vi "Create DatabaseTable.vi"() -> ()   [LabVIEW 2018]
doc: "This example allows you to perform several tasks on a database named LabVIEW.mdb located in the LabVIEW examples>>database directory.\n\nOperations include creating a table, creating a table and inserting data into named fields, creating a table and inserting data into generically named fields, or deleting a table."
uses:
  <vilib>/addons/database/Auxilliary.llb/DB Tools Column Info.ctl
  <vilib>/addons/database/Auxilliary.llb/DB Tools DataTypes.ctl
  <vilib>/addons/database/Connection.llb/DB Tools Open Connec (Path).vi
  <vilib>/addons/database/NI_Database_API.lvlib
panel:
  in  "sample data":T1={"String"="This is a test string", "Numeric"=101, "Numeric 2"=3.14}
  in  "column information":T2[](array[typedef])=[{"column name"="stringcol", "data type"=enum."String", "size"=50, "allow null?"=FALSE}, {"column name"="intcol", "data type"=enum."Long (I32)", "size"=0, "allow null?"=TRUE}, {"column name"="doublecol", "data type"=enum."Double (DBL)", "size"=0, "allow null?"=TRUE}]
  in  "Function":u16(ring) items=["Create Only", "Create and Insert (With Names)", "Create and Insert (Generic Names)", "Delete Table"]
  in  "Table":string="createtable"
  # "Overview: Demonstrates how to perform several tasks on a database.\nRequirements: Database Connectivity Toolkit\nInstructions:\n1. Select one of the 'Create' operations in the Function ring.\n2. Run the VI. The database table will be updated.\n3. Select another 'Create' operation and run the VI again.\n4. Select the 'Delete Table' operation and run the VI to remove the table from the database."
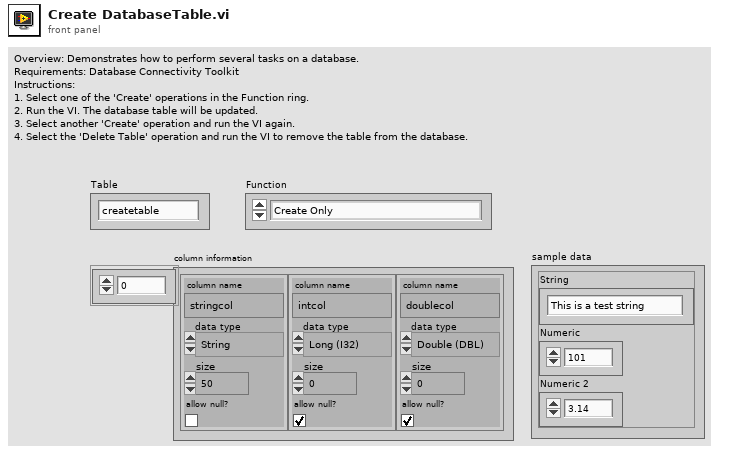
[diagram p1: front panel]
types:
  T1 = cluster{"String":string, "Numeric":i32, "Numeric 2":dbl}
  T2 = typedef "NI_Database_API.lvlib/DB Tools Column Info.ctl" = cluster{"column name":string, "data type":T3, "size":i32, "allow null?":bool}
  T3 = typedef "NI_Database_API.lvlib/DB Tools DataTypes.ctl" = enum16{"String", "Long (I32)", "Single (SGL)", "Double (DBL)", "Date/Time", "Binary"}
  T4 = typedef "NI_Database_API.lvlib/Conn ObjectReference.ctl" = refnum<k1>
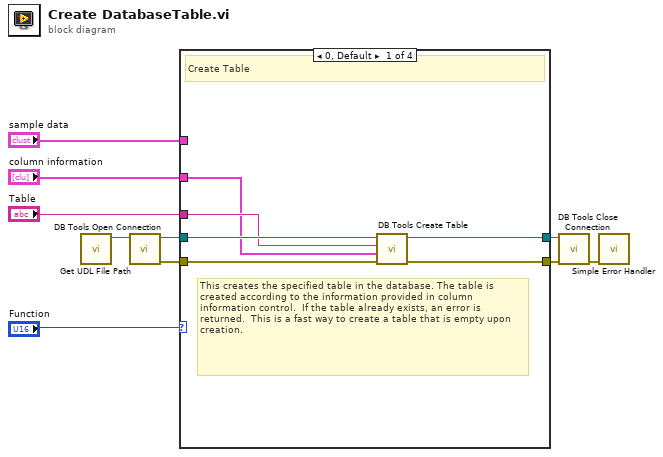
[diagram p0: block diagram]
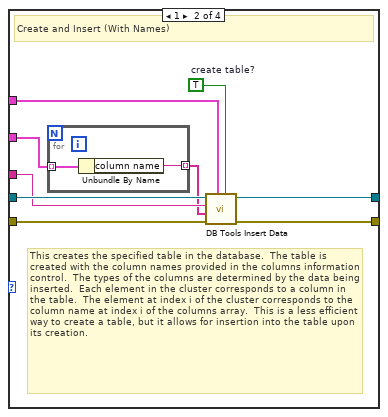
[diagram p2: hidden frame]
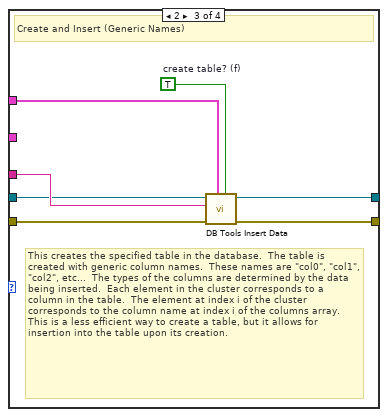
[diagram p3: hidden frame]
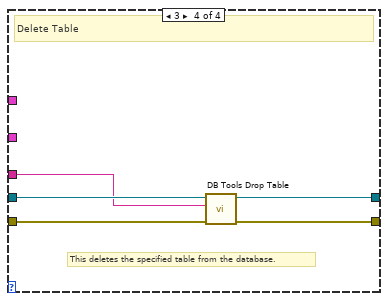
[diagram p4: hidden frame]
diagram:
  n1 = call "Get UDL File Path.vi"() -> ("UDL file path"=w10:path)  [unwired: 11 in]
  n2 = call-poly <vilib>:"DB Tools Open Connection.vi"("connection information"=w10) -> ("error out"=w5:errorcluster, "connection reference"=w6:T4)  [unwired: 7 in]
  n3 = case shown="0, Default" "Function" {
    tunnel: w6 -> [w16 w25 w29 w39]
    tunnel: w5 -> [w15 w22 w30 w38]
    tunnel: "Table" -> [w14 w19 w31 w35]
    tunnel: [w13 w20 w32 w37] -> w8
    tunnel: [w12 w21 w34 w36] -> w7
    tunnel: "sample data" -> [_ w23 w28 _]
    tunnel: "column information" -> [w11 w18 _ _]
    frame 0, Default {
      # "This creates the specified table in the database. The table is created according to the information provided in column information control.  If the table already exists, an error is returned.  This is a fast way to create a table that is empty upon creation."
      # "Create Table"
      n4 = call <vilib>:"DB Tools Create Table.vi"("error in (no error)"=w15, "column information"=w11, "table"=w14, "connection reference"=w16) -> ("error out"=w12:errorcluster, "connection reference out"=w13:T4)  [unwired: 4 in]
    }
    frame 1 {
      w24 = TRUE  # create table?
      # "This creates the specified table in the database.  The table is created with the column names provided in the columns information control.  The types of the columns are determined by the data being inserted.  Each element in the cluster corresponds to a column in the table.  The element at index i of the cluster corresponds to the column name at index i of the columns array.  This is a less efficient way to create a table, but it allows for insertion into the table upon its creation."
      # "Create and Insert (With Names)"
      n5 = for {
        tunnel: w18 -> [w27] mode=indexing
        tunnel: [w26] -> w17 mode=indexing
        n6 = Unbundle By Name(w27) -> ("column name"=w26:string)
      }
      n7 = call <vilib>:"DB Tools Insert Data.vi"("create table? (F)"=w24, "data"=w23, "error in (no error)"=w22, "columns"=w17, "table"=w19, "connection reference"=w25) -> ("error out"=w21:errorcluster, "connection reference out"=w20:T4)  [unwired: 4 in]
    }
    frame 2 {
      w33 = TRUE  # create table? (f)
      # "This creates the specified table in the database.  The table is created with generic column names.  These names are \"col0\", \"col1\", \"col2\", etc...  The types of the columns are determined by the data being inserted.  Each element in the cluster corresponds to a column in the table.  The element at index i of the cluster corresponds to the column name at index i of the columns array.  This is a less efficient way to create a table, but it allows for insertion into the table upon its creation."
      # "Create and Insert (Generic Names)"
      n8 = call <vilib>:"DB Tools Insert Data.vi"("create table? (F)"=w33, "data"=w28, "error in (no error)"=w30, "table"=w31, "connection reference"=w29) -> ("error out"=w34:errorcluster, "connection reference out"=w32:T4)  [unwired: 5 in]
    }
    frame 3 {
      # "This deletes the specified table from the database."
      # "Delete Table"
      n9 = call <vilib>:"DB Tools Drop Table.vi"("error in (no error)"=w38, "table"=w35, "connection reference"=w39) -> ("error out"=w36:errorcluster, "connection reference out"=w37:T4)  [unwired: 5 in]
    }
  }
  n10 = call <vilib>:"DB Tools Close Connection.vi"("error in (no error)"=w7, "connection reference"=w8) -> ("error out"=w3:errorcluster)  [unwired: 5 in]
  n11 = call <vilib>:"Simple Error Handler.vi"("error in (no error)"=w3) -> ()  [unwired: 4 in, 5 out]
